vi "Load Value.vi"(8 "Load Cell":dbl format="%0.03f", 10 "String in":refnum<vi>) -> ()   [LabVIEW 2020]
uses:
  Galobal variable_TI.vi
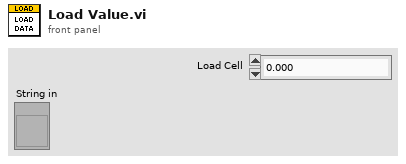
[diagram p1: front panel]
types:
  T1 = cluster{"MaxLoad ":dbl, "Min Load":dbl, "MaxDistance(mm)":dbl, "Min Distance(mm)":dbl, "Load Offset":dbl, "Model":string, "Difusser Code":string, "TFT Code ":string, "LVDT Offset":dbl}
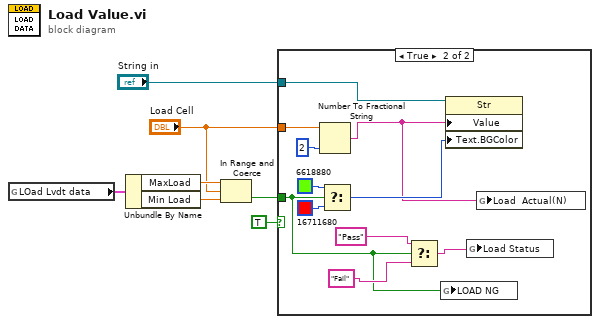
[diagram p0: block diagram]
diagram:
  n1 = global read "Galobal variable_TI.vi" "LOad Lvdt data"() -> (w6:T1)
  n2 = Unbundle By Name(w6) -> ("MaxLoad"=w5:dbl, "Min Load"=w4:dbl)
  n3 = In Range and Coerce(upper limit=w5, x="Load Cell", lower limit=w4) -> (In Range?=w7:bool)  [unwired: 1 out]
  n4 = case shown="True" TRUE {
    tunnel: w7 -> [_ w9]
    tunnel: "Load Cell" -> [_ w14]
    tunnel: "String in" -> [_ w13]
    frame False {
    }
    frame True {
      n5 = Number To Fractional String(number=w14, precision (6)=i16 2) -> (F-format string=w8:string)  [unwired: 2 in]
      n6 = Select(t=u32 6618880, s=w9, f=u32 16711680) -> (s? t:f=w18:u32)
      n7 = Select(t="Pass", s=w9, f="Fail") -> (s? t:f=w10:string)
      n8 = global write "Galobal variable_TI.vi" "LOAD NG"(w9) -> ()
      n9 = property class="Str"(reference=w13, "Value"=w8, "Text.BGColor"=w18) -> ()  [unwired: 1 in, 2 out]
      n10 = global write "Galobal variable_TI.vi" "Load Status"(w10) -> ()
      n11 = global write "Galobal variable_TI.vi" "Load  Actual(N)"(w8) -> ()
    }
  }
